vi "Set both gates.vi"(4 "Error In":errorcluster caption="Error", 5 "VISA resource name":refnum<visa-resource-name>, 6 "Set Delay?":bool, 7 "Set Width?":bool, 8 "gatedelayoffsetB":dbl[unit] caption="Gate B Delay", 9 "gatedelayoffsetA":dbl[unit] caption="Gate A Delay", 10 "Gate B Width":dbl[unit], 11 "Gate A Width":dbl[unit]) -> (0 "Error Out":errorcluster, 3 "VISA resource name out":refnum<visa-resource-name>)   [LabVIEW 2015, in "SR400.lvlib"]
uses:
  SR400.lvlib
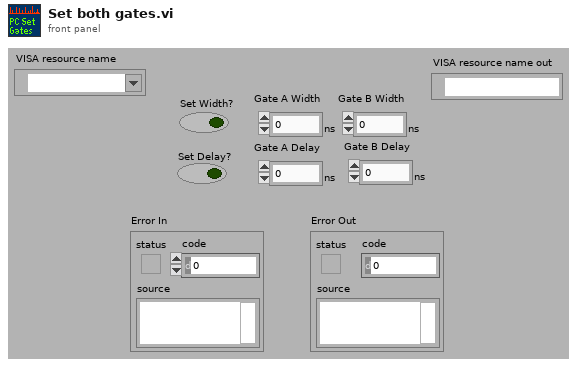
[diagram p1: front panel]
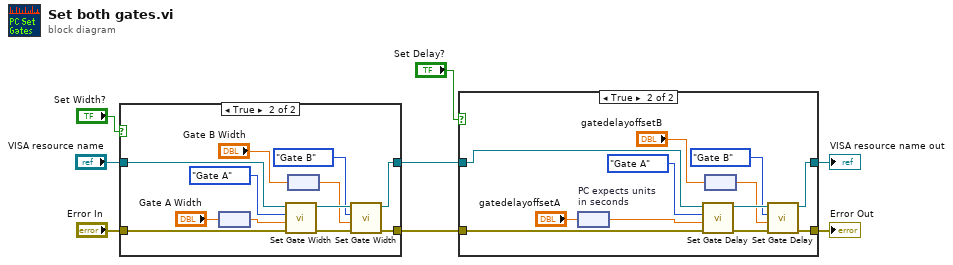
[diagram p0: block diagram]
diagram:
  n1 = case shown="True" "Set Width?" {
    tunnel: "Error In" -> [w10 w17]
    tunnel: [w10 w12] -> w5
    tunnel: "VISA resource name" -> [w9 w20]
    tunnel: [w9 w11] -> w4
    frame False {
    }
    frame True {
      n2 = node("Gate A Width") -> (w18:dbl)
      n3 = call "Set Gate Width.vi"("error in (no error)"=w17, "Width (def: 0 s)"=w18, "Gate (def: A)"=enum16{"Gate A", "Gate B"}."Gate A" ("i (0)"), "VISA resource name"=w20) -> ("error out"=w15:errorcluster, "VISA resource name out"=w16:refnum<visa-resource-name>)  [unwired: 6 out]
      n4 = node("Gate B Width") -> (w13:dbl)
      n5 = call "Set Gate Width.vi"("error in (no error)"=w15, "Width (def: 0 s)"=w13, "Gate (def: A)"=enum16{"Gate A", "Gate B"}."Gate B" ("i (0)"), "VISA resource name"=w16) -> ("error out"=w12:errorcluster, "VISA resource name out"=w11:refnum<visa-resource-name>)  [unwired: 6 out]
    }
  }
  n6 = case shown="True" "Set Delay?" {
    tunnel: w5 -> [w23 w31]
    tunnel: w4 -> [w24 w34]
    tunnel: [w24 w29] -> w2
    tunnel: [w23 w27] -> w1
    frame False {
    }
    frame True {
      n7 = node "PC expects units\nin seconds"("gatedelayoffsetA") -> (w32:dbl)
      n8 = call "Set Gate Delay.vi"("error in (no error)"=w31, "Delay (Def: 0 s)"=w32, "Gate (Def: A)"=enum16{"Gate A", "Gate B"}."Gate A" ("i (0)"), "VISA resource name"=w34) -> ("error out"=w28:errorcluster, "VISA resource name out"=w30:refnum<visa-resource-name>)  [unwired: 6 out]
      n9 = node("gatedelayoffsetB") -> (w25:dbl)
      n10 = call "Set Gate Delay.vi"("error in (no error)"=w28, "Delay (Def: 0 s)"=w25, "Gate (Def: A)"=enum16{"Gate A", "Gate B"}."Gate B" ("i (0)"), "VISA resource name"=w30) -> ("error out"=w27:errorcluster, "VISA resource name out"=w29:refnum<visa-resource-name>)  [unwired: 6 out]
    }
  }
  "Error Out" <- w1
  "VISA resource name out" <- w2
